vi "OpenDevice.vi"(8 "error in (no error)":errorcluster, 10 "Def-OpenDevice":T1, 11 "CAN-NI in":refnum<class "CAN-NI.lvclass">) -> (0 "error out":errorcluster, 3 "CAN-NI out":refnum<class "CAN-NI.lvclass">)   [LabVIEW 2019, in "CAN-NI.lvlib" / "CAN-NI.lvclass"]
uses:
  CAN-NI.lvclass
  CAN-Interface/TypeDef/Def-OpenDevice.ctl
  CAN-Interface/Class-Interface.lvclass
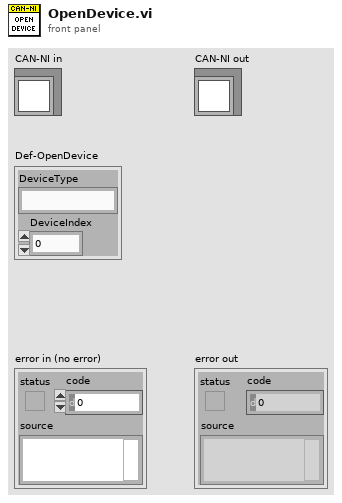
[diagram p1: front panel]
types:
  T1 = typedef "CAN-Interface.lvlib/Class-Interface.lvclass/Def-OpenDevice.ctl" = cluster{"DeviceType":string, "DeviceIndex":u32}
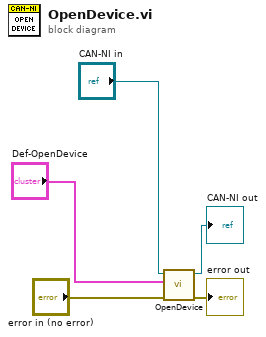
[diagram p0: block diagram]
diagram:
  n1 = call-parent "OpenDevice.vi"("error in (no error)"="error in (no error)", "Def-OpenDevice"="Def-OpenDevice", "Class-Interface in"="CAN-NI in") -> ("error out"=→"error out":errorcluster, "Class-Interface out"=→"CAN-NI out":refnum<class "CAN-NI.lvclass">)  [unwired: 7 in]
